vi "Open IPS.vi"(8 "error in (no error)":errorcluster, 11 "Instrument.Oxford1820 in":refnum<class "Instrument.OxfordVRM.lvclass">) -> (0 "error out":errorcluster, 3 "Instrument.Oxford1820 out":refnum<class "Instrument.OxfordVRM.lvclass">)   [LabVIEW 2016, in "Instrument.OxfordVRM.lvclass"]
uses:
  Instrument.OxfordVRM.lvclass
  <instrlib>/Mercury iXX/Mercury iXX.lvlib
  <instrlib>/Mercury iXX/Public/Libraries/System/Open/Open System.vi
  <instrlib>/Mercury iXX/Public/Libraries/System.lvlib
  <instrlib>/Mercury iXX/Public/Controls/Comms Transport Layer.ctl
  <instrlib>/Mercury iXX/Public/Libraries/System/Read/Catalogue (Read).vi
  <instrlib>/Mercury iXX/Public/Libraries/Magnet/Controls/Identifier.ctl
  <instrlib>/Mercury iXX/Public/Libraries/Magnet.lvlib
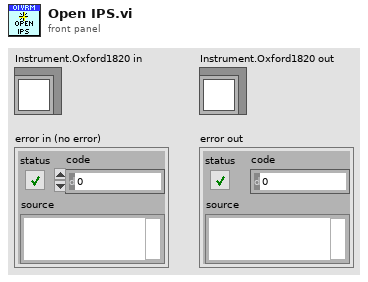
[diagram p1: front panel]
types:
  T1 = typedef "Mercury iXX.lvlib/Magnet.lvlib/Identifier.ctl" = string
  T2 = typedef "Mercury iXX.lvlib/Comms Transport Layer.ctl" = enum16{"Ethernet TCP/IP", "USB", "ISOBus - RS-232", "GPIB"}
  T3 = typedef "Mercury iXX.lvlib/Mercury Reference.ctl" = cluster{"Comms":refnum<visa-resource-name>, "Device ID":string[], "Comms Layer":T2, "Command":string, "Query reference":T4}
  T4 = typedef "Mercury iXX.lvlib/Query Dynamic Reference.ctl" = refnum<vi>
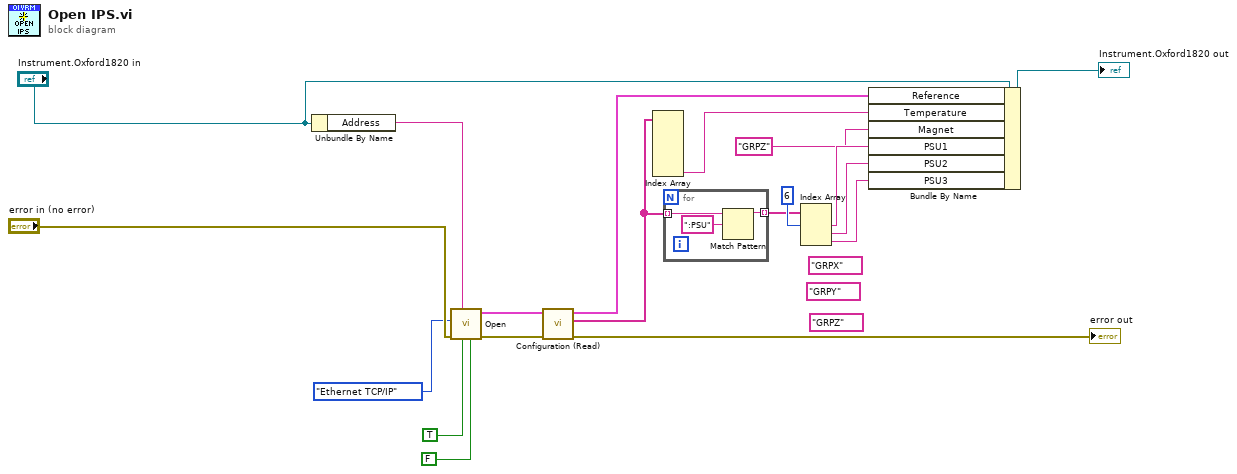
[diagram p0: block diagram]
diagram:
  (unwired) T1 "GRPZ" ("Device Identifier 2")
  (unwired) T1 "GRPY" ("Device Identifier 2")
  (unwired) T1 "GRPX" ("Device Identifier 2")
  n1 = Unbundle By Name("Instrument.Oxford1820 in") -> ("Address"=w4:string)
  n2 = call-poly <instrlib>:"Open.vi"("Clear Previous Connections (False)"=FALSE, "ID Query (True)"=TRUE, "IP Address"=w4, "error in (no error)"="error in (no error)", "Comms Layer"=Comms_Transport_Layer."Ethernet TCP/IP") -> ("error out"=w6:errorcluster, "Mercury Reference Out"=w7:T3)  [unwired: 2 in, 3 out]
  n3 = call-poly <instrlib>:"Configuration (Read).vi"("error in"=w6, "Mercury Reference In"=w7) -> ("error out"=→"error out":errorcluster, "Devices"=w13:string[], "Mercury Reference Out"=w9:T3)  [unwired: 1 in, 6 out]
  n4 = Index Array(array=w13) -> (element #6=w1:string)  [unwired: 6 in, 5 out]
  n5 = for {
    tunnel: w13 -> [w21] mode=indexing
    tunnel: [w20] -> w11 mode=indexing
    n6 = Match Pattern(string=w21, regular expression=":PSU") -> (before substring=w20:string)  [unwired: 1 in, 3 out]
  }
  n7 = Index Array(array=w11, index #1=6 ("index")) -> (element #1=w15:string, element #2=w16:string, element #3=w17:string)  [unwired: 2 in]
  n8 = Bundle By Name(cluster="Instrument.Oxford1820 in", "Reference"=w9, "Temperature"=w1, "Magnet"="GRPZ" ("IPS.Devices.Magnet (GRPZ)"), "PSU1"=w15, "PSU2"=w16, "PSU3"=w17) -> (→"Instrument.Oxford1820 out":refnum<class "Instrument.OxfordVRM.lvclass">)
